vi "Format to TmeStamp.vi"(8 "error in":errorcluster, 11 "String":string) -> (0 "error out":errorcluster, 3 "Time Stamp":timestamp format="%<%I:%M:%S%3u %p\n%m/%d/%Y>T")   [LabVIEW 2018, in "Data Operations.lvlib"]
uses:
  Data Operations.lvlib
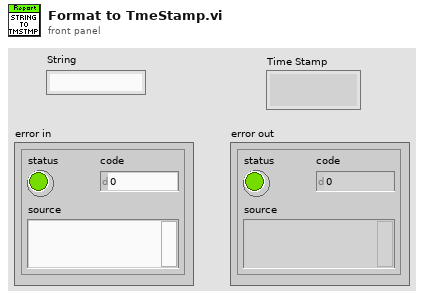
[diagram p1: front panel]
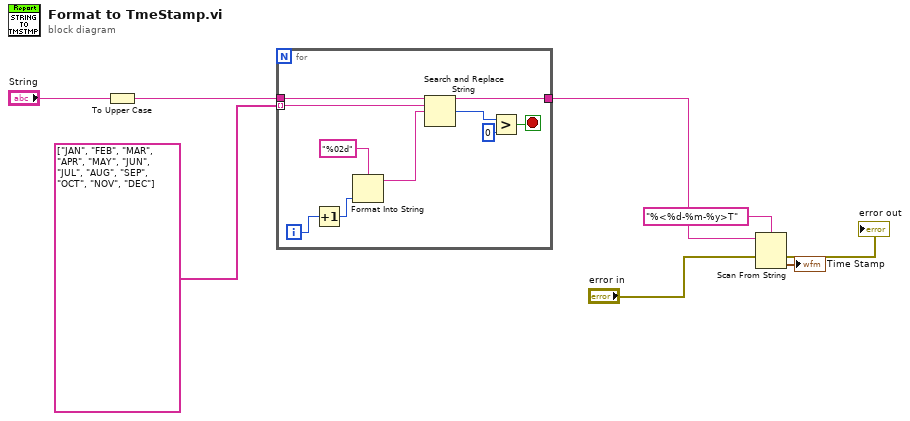
[diagram p0: block diagram]
diagram:
  n1 = To Upper Case(1:"String") -> (0:w1:string)
  n2 = for {
    tunnel: w1 -> [w18]
    tunnel: string[] ["JAN", "FEB", "MAR", "APR", "MAY", "JUN", "JUL", "AUG", "SEP", "OCT", "NOV", "DEC"] -> [w17] mode=indexing
    tunnel: [w9] -> w4
    i -> [w16]
    stop <- w10 stop-if-true
    n3 = Increment(x=w16) -> (x+1=w15:i32)
    n4 = Format Into String(format string="%02d", w15) -> (resulting string=w13:string)  [unwired: 2 in, 1 out]
    n5 = Search and Replace String(input string=w18, search string=w17, replace string=w13) -> (result string=w9:string, number of replacements=w12:i32)  [unwired: 5 in, 2 out]
    n6 = Greater?(x=w12, y=0) -> (0:w10:bool)
  }
  n7 = Scan From String "Scan From String"(format string="%<%d-%m-%y>T", input string=w4, error in="error in") -> (error out=→"error out":errorcluster, output 1=→"Time Stamp":timestamp)  [unwired: 2 in, 2 out]
